vi "Load Scale And Calibration.vi"(6 "Database?":bool, 7 "Database Data":T1={"Server"="127.0.0.1", "Port"=3306, "UserID"="root", "Password"="password", "Database"="737_rpi"}, 8 "error in (no error)":errorcluster, 10 "polynomial order":i32=5, 11 "appended path":path) -> (0 "error out":errorcluster, 1 "all rows":dbl[][](array[numeric]), 2 "intercept":dbl, 3 "slope":dbl, 4 "Calibration Info":string, 5 "Polynomial Coefficients":dbl[](array[numeric]) format="%#_15g")   [LabVIEW 2017]
uses:
  MySQL NET Database VIs/Controls/Database Connection Data.ctl
  MySQL NET Database VIs/Controls/Database Command.ctl
  <vilib>/Utility/file.llb/Read From Spreadsheet File (DBL).vi
  <vilib>/Analysis/NI_AALPro.lvlib
  MySQL NET Database VIs/VIs to Interface LabVIEW and MySQL dotNET Connector.lvlib
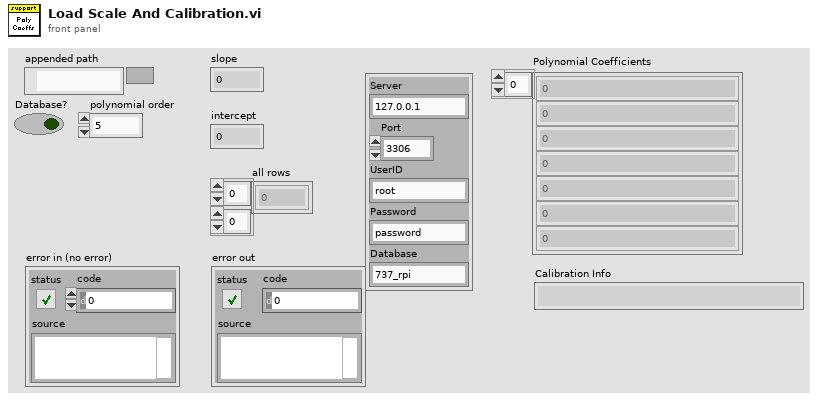
[diagram p1: front panel]
types:
  T1 = typedef "VIs to Interface LabVIEW and MySQL dotNET Connector.lvlib/Database Connection Data.ctl" = cluster{"Server":string, "Port":u32, "UserID":string, "Password":string, "Database":string}
  T2 = typedef "VIs to Interface LabVIEW and MySQL dotNET Connector.lvlib/Database Command.ctl" = enum16{"Insert", "Update", "Select All", "Delete Entry", "Drop Table", "SQL Command", "Select", "Get Column Info", "Select Column"}
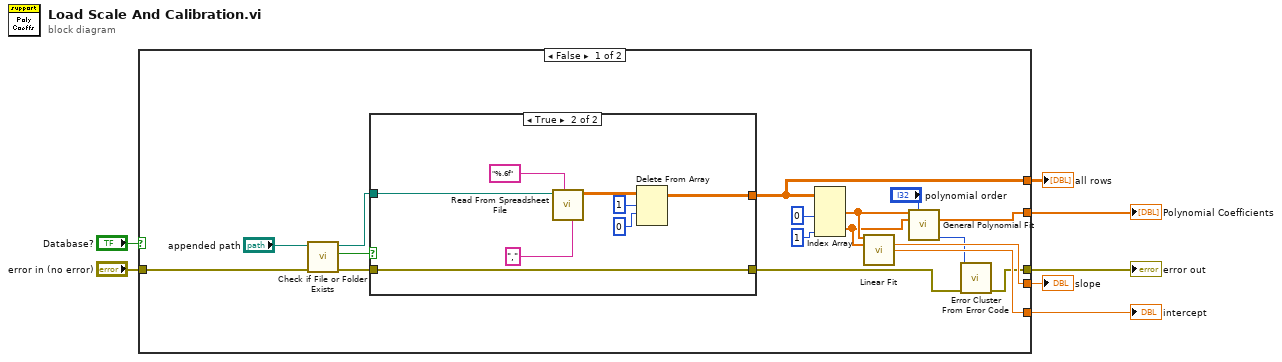
[diagram p0: block diagram]
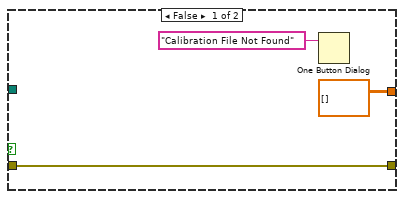
[diagram p2: hidden frame]
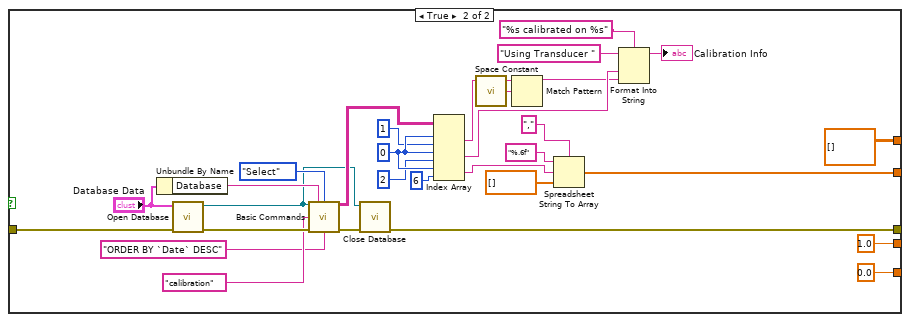
[diagram p3: hidden frame]
diagram:
  n1 = case shown="False" "Database?" {
    tunnel: [w17 dbl[][] [] ("all rows")] -> w7
    tunnel: [w9 w47] -> w6
    tunnel: "error in (no error)" -> [w21 w65]
    tunnel: [w13 1.0 ("slope")] -> w3
    tunnel: [w12 0.0 ("intercept")] -> w2
    tunnel: [w11 w49] -> w1
    frame False {
      n2 = call <vilib>:"Check if File or Folder Exists.vi"("error in (no error)"=w21, "path"="appended path") -> ("error out"=w22:errorcluster, "file or folder exists?"=w23:bool, "dup path"=w24:path)  [unwired: 7 in]
      n3 = case shown="True" w23 {
        tunnel: w22 -> [w27 w35]
        tunnel: [w27 w35] -> w8
        tunnel: w24 -> [_ w34]
        tunnel: [dbl[][] [] ("all rows") w28] -> w17
        frame False {
          n4 = One Button Dialog(message="Calibration File Not Found") -> ()  [unwired: 1 in, 1 out]
        }
        frame True {
          n5 = call-poly <vilib>:"Read From Spreadsheet File.vi"("delimiter (\\t)"="," ("delimiter (\\t)"), "format (%.3f)"="%.6f", "file path (dialog if empty)"=w34) -> ("all rows"=w31:dbl[][])  [unwired: 4 in, 4 out]
          n6 = Delete From Array(array=w31, length=1, index (row)=0) -> (array with subset deleted=w28:dbl[][])  [unwired: 1 in, 1 out]
        }
      }
      n7 = Index Array(array=w17, index (col) #1=0 ("disabled index (col)"), index (col) #2=1 ("index (col)")) -> (element #1=w15:dbl[], element #2=w14:dbl[])  [unwired: 2 in]
      n8 = call <vilib>:"Linear Fit.vi"("Y"=w15, "X"=w14) -> ("slope"=w13:dbl, "intercept"=w12:dbl)  [unwired: 9 in, 3 out]
      n9 = call <vilib>:"General Polynomial Fit.vi"("Y"=w15, "polynomial order"="polynomial order", "X"=w14) -> ("Polynomial Coefficients"=w11:dbl[], "error"=w10:i32)  [unwired: 9 in, 2 out]
      n10 = call <vilib>:"Error Cluster From Error Code.vi"("error in (no error)"=w8, "error code (0)"=w10) -> ("error out"=w9:errorcluster)  [unwired: 7 in]
    }
    frame True {
      w45 = 0 ("index (row)")
      n11 = Unbundle By Name("Database Data") -> ("Database"=w62:string)
      n12 = call "Open Database.vi"("error in (no error)"=w65, 11:"Database Data") -> ("error out"=w64:errorcluster, ".Net dbase ref"=w46:refnum<k24>)  [unwired: 8 in]
      n13 = call "Basic Commands.vi"(".NET Refnum in"=w46, "Database"=w62, "Database Command"=Database_Command."Select", "Table"="calibration", "error in (no error)"=w64, "Condition"="ORDER BY `Date` DESC") -> ("Data Array"=w58:string[][], "error out"=w48:errorcluster)  [unwired: 7 in, 1 out]
      n14 = call "Close Database.vi"("error in (no error)"=w48, ".NET Refnum in"=w46) -> ("error out"=w47:errorcluster)  [unwired: 9 in]
      n15 = Index Array(array=w58, index (row) #1=w45, index (col) #1=1 ("disabled index (col)"), index (row) #2=w45, index (col) #2=2 ("disabled index (col)"), index (row) #3=w45, index (col) #3=6 ("disabled index (col)")) -> (element #1=w37:string, element #2=w39:string, element #3=w53:string)
      n16 = call <vilib>:"Space Constant.vi"() -> ("String"=w38:string)
      n17 = Match Pattern(string=w37, regular expression=w38) -> (before substring=w36:string)  [unwired: 1 in, 3 out]
      n18 = Spreadsheet String To Array(delimiter (Tab)=",", format string="%.6f", spreadsheet string=w53, array type (2D Dbl)=dbl[] [] ("Polynomial Coefficients")) -> (array=w49:dbl[])
      n19 = Format Into String(format string="%s calibrated on %s", initial string="Using Transducer ", w39, w36) -> (resulting string=→"Calibration Info":string)  [unwired: 1 in, 1 out]
    }
  }
  "all rows" <- w7
  "intercept" <- w2
  "slope" <- w3
  "error out" <- w6
  "Polynomial Coefficients" <- w1
